vi "PTScanner.DIM Update.vi"(0 "i ref in":refnum<vi>, 1 "serviceName":string, 2 "quality":i32, 3 "Time Stamp":dbl, 4 "data":i8[](array[numeric]), 5 "error in (no error)":errorcluster, 7 "no link":bool, 9 "typeDescriptor":string) -> (14 "i ref out":refnum<vi>, 19 "error out":errorcluster)   [LabVIEW 2014, in "PTScanner.lvlib"]
uses:
  PTScanner.lvlib
  _common/PTUtils/PTUtils.lvlib
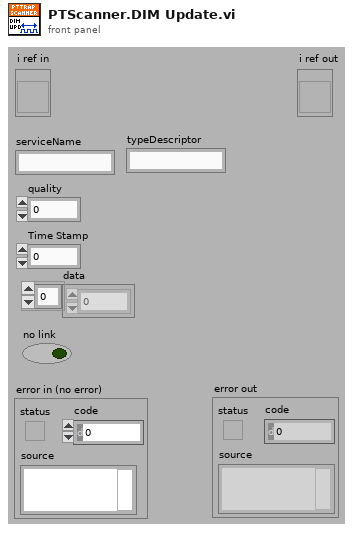
[diagram p1: front panel]
types:
  T1 = typedef "PTScanner.lvlib/PTScanner.i attribute.ctl" = cluster{"Object cmds":T2[], "Steps":cluster{"Finished":bool, "cmd setup":T3[]}[], "curStep":i32, "DIM IDs":cluster{"AllFinished":i32, "Finished":i32, "curStep":i32, "nofSteps":i32, "NomValues":i32[], "1D-Min":i32, "1D-Max":i32, "Dimensions":i32, "MaxDimensions":i32, "ScanedDeviceNames":i32[]}, "All Finished":bool, "DIMs in use":string[], "Running":bool, "Scan Delay":u32, "loop":bool, "Paused":bool, "Formed":bool}
  T2 = typedef "PTScanner.lvlib/PTScanner.obj parameters.ctl" = cluster{"object":string, "DIM address":string, "method":string, "data descriptor":string, "method parameters":cluster{"Name":string, "Descr":string, "Value":string, "Value?":bool}[], "Call Mode":enum16{"Simple DIM", "Synchronous"}, "actValue":dbl, "Centroid":dbl, "Minus Delta":dbl, "Plus Delta":dbl, "increment":dbl, "DIM Status":cluster{"no link":bool, "quality":i32, "Time Stamp":timestamp}, "range":dbl, "DIMChannelIndex":i32}
  T3 = typedef "PTScanner.lvlib/PTScanner.step obj parameters.ctl" = cluster{"obj index":i32, "nomValue":dbl, "fulfilled":bool}
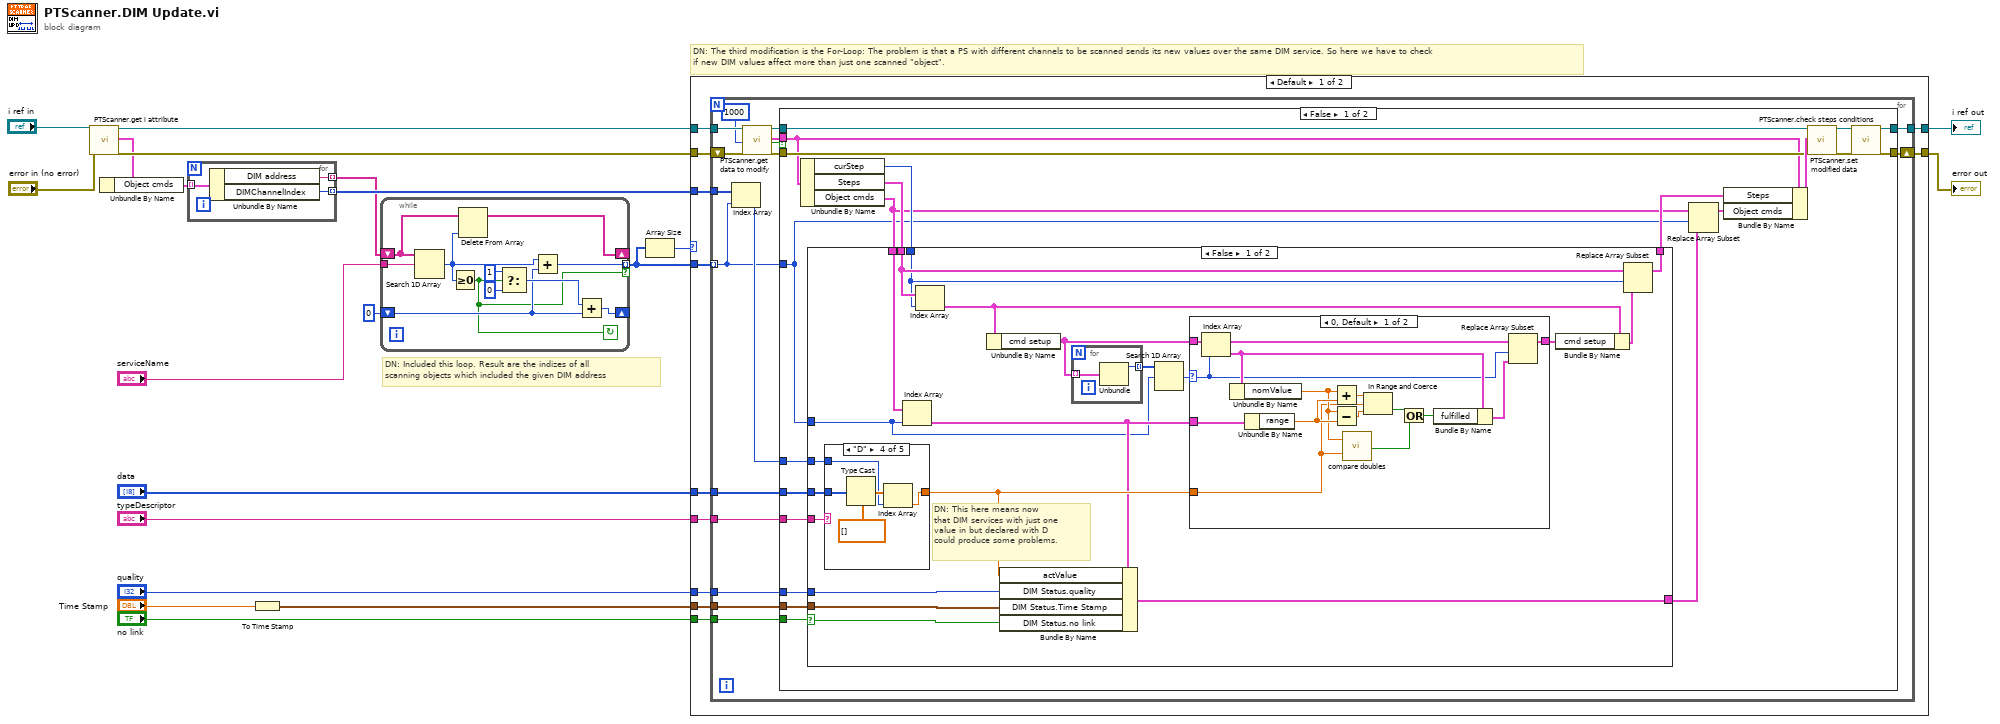
[diagram p0: block diagram]
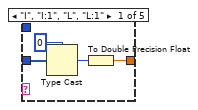
[diagram p3: hidden frame]
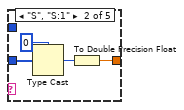
[diagram p4: hidden frame]
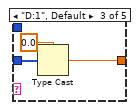
[diagram p5: hidden frame]
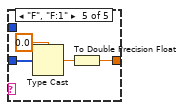
[diagram p6: hidden frame]
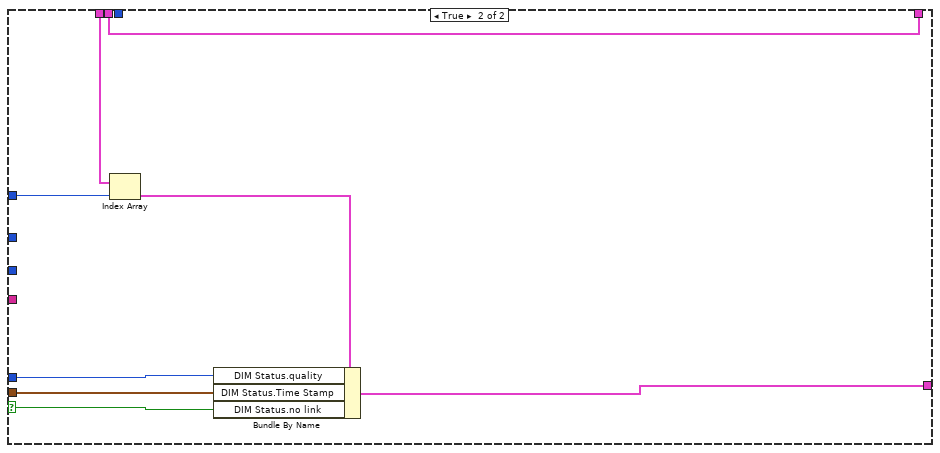
[diagram p7: hidden frame]
diagram:
  # "DN: The third modification is the For-Loop: The problem is that a PS with different channels to be scanned sends its new values over the same DIM service. So here we have to check\nif new DIM values affect more than just one scanned \"object\"."
  # "DN: Included this loop. Result are the indizes of all\nscanning objects which included the given DIM address"
  n1 = call "PTScanner.get i attribute.vi"("i ref in"="i ref in", "error in (no error)"="error in (no error)") -> ("i ref out"=w19:refnum<vi>, "i attribute"=w17:T1, "error out"=w18:errorcluster)  [unwired: 15 in]
  n2 = Unbundle By Name(w17) -> ("Object cmds"=w8:T2[])
  n3 = for {
    tunnel: w8 -> [w23] mode=indexing
    tunnel: [w22] -> w4 mode=indexing
    tunnel: [w21] -> w6 mode=indexing
    n4 = Unbundle By Name(w23) -> ("DIM address"=w22:string, "DIMChannelIndex"=w21:i32)
  }
  n5 = To Time Stamp(1:"Time Stamp") -> (0:w20:timestamp)
  n6 = while {
    tunnel: "serviceName" -> [w34]
    tunnel: [w26] -> w1 mode=indexing if=w24
    shift-right: [w32] -> _
    shift-left: w4 -> [w33]
    shift-right: [w28] -> _
    shift-left: 0 -> [w25]
    stop <- w24 continue-if-true
    n7 = Search 1D Array(1D array=w33, element=w34) -> (index of element=w27:i32)  [unwired: 1 in]
    n8 = Greater Or Equal To 0?(x=w27) -> (x >= 0?=w24:bool)
    n9 = Delete From Array(array=w33, index=w27) -> (array with subset deleted=w32:string[])  [unwired: 1 in, 1 out]
    n10 = Select(t=1, s=w24, f=0) -> (s? t:f=w29:i32)
    n11 = Add(x=w27, y=w25) -> (x+y=w26:i32)
    n12 = Add(x=w29, y=w25) -> (x+y=w28:i32)
  }
  n13 = Array Size(array=w1) -> (size(s)=w2:i32)
  n14 = case shown="Default" w2 {
    tunnel: [w45 w151] -> w10
    tunnel: [w44 w152] -> w16
    tunnel: "data" -> [w43 _]
    tunnel: "quality" -> [w42 _]
    tunnel: w20 -> [w41 _]
    tunnel: "no link" -> [w40 _]
    tunnel: w19 -> [w39 w152]
    tunnel: w18 -> [w38 w151]
    tunnel: "typeDescriptor" -> [w37 _]
    tunnel: w6 -> [w36 _]
    tunnel: w1 -> [w35 _]
    frame Default {
      n15 = for {
        tunnel: [w57] -> w44
        tunnel: w43 -> [w56]
        tunnel: w42 -> [w55]
        tunnel: w41 -> [w54]
        tunnel: w40 -> [w53]
        tunnel: w39 -> [w52]
        tunnel: w37 -> [w49]
        tunnel: w36 -> [w48]
        tunnel: w35 -> [w46] mode=indexing
        shift-right: [w58] -> w45
        shift-left: w38 -> [w50]
        n16 = Index Array(array=w48, index=w46) -> (element=w47:i32)
        n17 = call "PTScanner.get data to modify.vi"("i ref in"=w52, "ms timeout (10000)"=1000, "error in (no error)"=w50) -> ("i ref out"=w60:refnum<vi>, "i attribute"=w61:T1, "timed out"=w62:bool, "error out"=w59:errorcluster)  [unwired: 13 in]
        n18 = case shown="False" w62 {
          tunnel: w61 -> [w75 _]
          tunnel: w60 -> [w77 w149]
          tunnel: [w64 w150] -> w58
          tunnel: w59 -> [w78 w150]
          tunnel: [w65 w149] -> w57
          tunnel: w56 -> [w80 _]
          tunnel: w55 -> [w82 _]
          tunnel: w54 -> [w81 _]
          tunnel: w53 -> [w83 _]
          tunnel: w49 -> [w71 _]
          tunnel: w46 -> [w68 _]
          tunnel: w47 -> [w63 _]
          frame False {
            n19 = Unbundle By Name(w75) -> ("curStep"=w74:i32, "Steps"=w76:cluster{"Finished":bool, "cmd setup":T3[]}[], "Object cmds"=w70:T2[])
            n20 = case shown="False" w83 {
              selector: w83 -> [w99 w146]
              tunnel: w82 -> [w101 w148]
              tunnel: w81 -> [w100 w147]
              tunnel: w80 -> [w102 _]
              tunnel: w76 -> [w96 w142]
              tunnel: w74 -> [w94 _]
              tunnel: [w93 w142] -> w73
              tunnel: w71 -> [w103 _]
              tunnel: w70 -> [w98 w145]
              tunnel: [w91 w144] -> w69
              tunnel: w68 -> [w87 w143]
              tunnel: w63 -> [w84 _]
              frame False {
                # "DN: This here means now\nthat DIM services with just one\nvalue in but declared with D\ncould produce some problems."
                n21 = case shown="\"D\"" w103 {
                  tunnel: w102 -> [w123 w127 w130 w136 w139]
                  tunnel: [w121 w125 w129 w133 w137] -> w89
                  tunnel: w84 -> [_ _ _ w132 _]
                  frame "I", "I:1", "L", "L:1" {
                    n22 = Type Cast(type=0, x=w123) -> (*(type *) &x=w122:i32)
                    n23 = To Double Precision Float(number=w122) -> (double precision float=w121:dbl)
                  }
                  frame "S", "S:1" {
                    n24 = Type Cast(type=i16 0, x=w127) -> (*(type *) &x=w126:i16)
                    n25 = To Double Precision Float(number=w126) -> (double precision float=w125:dbl)
                  }
                  frame "D:1", Default {
                    n26 = Type Cast(type=0.0, x=w130) -> (*(type *) &x=w129:dbl)
                  }
                  frame "D" {
                    n27 = Type Cast(type=dbl[] [], x=w136) -> (*(type *) &x=w134:dbl[])
                    n28 = Index Array(array=w134, index=w132) -> (element=w133:dbl)
                  }
                  frame "F", "F:1" {
                    n29 = Type Cast(type=sgl 0.0, x=w139) -> (*(type *) &x=w138:sgl)
                    n30 = To Double Precision Float(number=w138) -> (double precision float=w137:dbl)
                  }
                }
                n31 = Index Array(array=w98, index=w87) -> (element=w88:T2)
                n32 = Index Array(array=w96, index=w94) -> (element=w97:cluster{"Finished":bool, "cmd setup":T3[]})
                n33 = Unbundle By Name(w97) -> ("cmd setup"=w90:T3[])
                n34 = Bundle By Name(cluster=w88, "actValue"=w89, "DIM Status.quality"=w101, "DIM Status.Time Stamp"=w100, "DIM Status.no link"=w99) -> (w91:T2)
                n35 = for {
                  tunnel: w90 -> [w120] mode=indexing
                  tunnel: [w119] -> w92 mode=indexing
                  n36 = Unbundle(w120) -> ("obj index"=w119:i32)  [unwired: 2 out]
                }
                n37 = Search 1D Array(1D array=w92, element=w87) -> (index of element=w85:i32)  [unwired: 1 in]
                n38 = case shown="0, Default" w85 {
                  selector: w85 -> [w104 _]
                  tunnel: w90 -> [w109 w118]
                  tunnel: w89 -> [w107 _]
                  tunnel: w88 -> [w106 _]
                  tunnel: [w105 w118] -> w86
                  frame 0, Default {
                    n39 = Index Array(array=w109, index=w104) -> (element=w110:T3)
                    n40 = Unbundle By Name(w110) -> ("nomValue"=w116:dbl)
                    n41 = Unbundle By Name(w106) -> ("range"=w117:dbl)
                    n42 = Add(x=w116, y=w117) -> (x+y=w114:dbl)
                    n43 = Subtract(x=w116, y=w117) -> (x-y=w115:dbl)
                    n44 = call "compare doubles.vi"("base value"=w116, "value to compare"=w107) -> ("Equal"=w112:bool)  [unwired: 17 in]
                    n45 = In Range and Coerce(upper limit=w114, x=w107, lower limit=w115) -> (In Range?=w113:bool)  [unwired: 1 out]
                    n46 = Or(x=w113, y=w112) -> (x .or. y?=w111:bool)
                    n47 = Bundle By Name(cluster=w110, "fulfilled"=w111) -> (w108:T3)
                    n48 = Replace Array Subset(array=w109, new element=w108, index=w104) -> (w105:T3[])
                  }
                  frame -1 {
                  }
                }
                n49 = Bundle By Name(cluster=w97, "cmd setup"=w86) -> (w95:cluster{"Finished":bool, "cmd setup":T3[]})
                n50 = Replace Array Subset(array=w96, new element=w95, index=w94) -> (w93:cluster{"Finished":bool, "cmd setup":T3[]}[])
              }
              frame True {
                n51 = Index Array(array=w145, index=w143) -> (element=w141:T2)
                n52 = Bundle By Name(cluster=w141, "DIM Status.quality"=w148, "DIM Status.Time Stamp"=w147, "DIM Status.no link"=w146) -> (w144:T2)
              }
            }
            n53 = Replace Array Subset(array=w70, new element=w69, index=w68) -> (w72:T2[])
            n54 = Bundle By Name(cluster=w75, "Steps"=w73, "Object cmds"=w72) -> (w79:T1)
            n55 = call "PTScanner.set modified data.vi"("i ref in"=w77, "CLASS.i attribute"=w79, "error in (no error)"=w78) -> ("i ref out"=w66:refnum<vi>, "error out"=w67:errorcluster)  [unwired: 15 in]
            n56 = call "PTScanner.check steps conditions.vi"("i ref in"=w66, "error in (no error)"=w67) -> ("i ref out"=w65:refnum<vi>, "error out"=w64:errorcluster)  [unwired: 14 in, 2 out]
          }
          frame True {
          }
        }
      }
    }
    frame 0 {
    }
  }
  "i ref out" <- w16
  "error out" <- w10
